vi "Not sure.vi"(6 "offset of match":i32, 7 "String":string, 9 "offset of match 2":i32, 10 "Plot Sizes":i32[](array[numeric]), 11 "String 2":string) -> (3 "Array":i32[](array[numeric]))   [LabVIEW 2021]
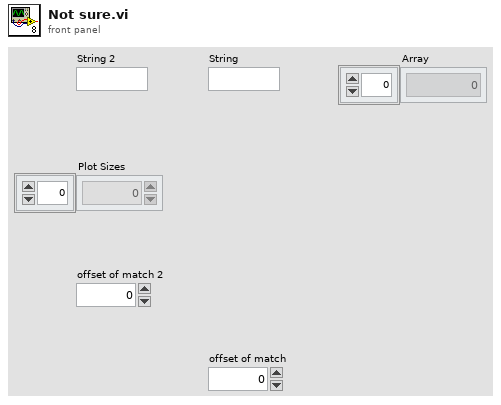
[diagram p1: front panel]
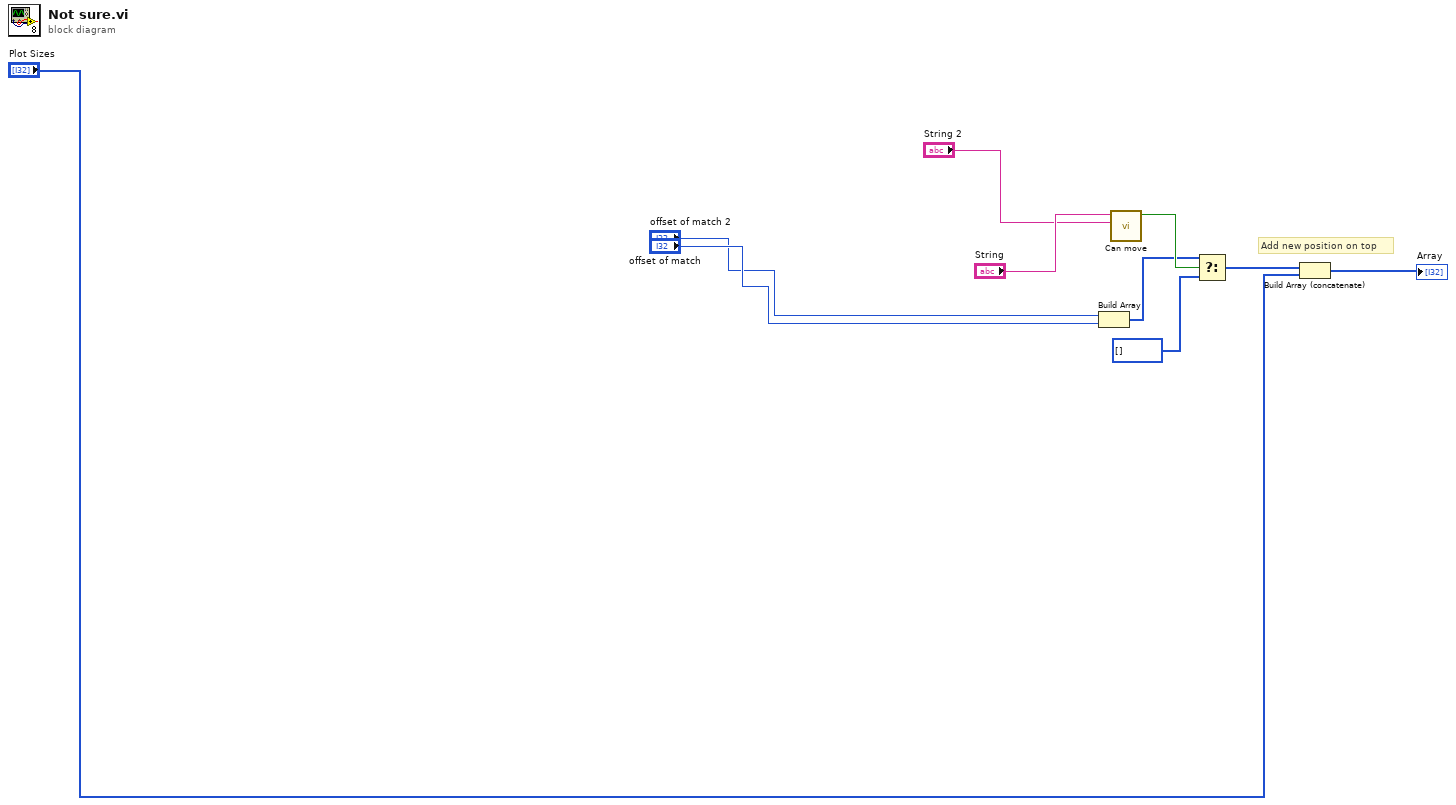
[diagram p0: block diagram]
diagram:
  # "Add new position on top"
  n1 = Build Array("offset of match 2", "offset of match") -> (w6:i32[])
  n2 = call "Can move"("Current letter"="String 2", "New letter"="String") -> ("Can move"=w7:bool)  [unwired: 9 in]
  n3 = Select(t=w6, s=w7, f=i32[] []) -> (s? t:f=w9:i32[])
  n4 = Build Array (concatenate)(w9, "Plot Sizes") -> (→"Array":i32[])
